vi "Create.vi"(8 "error in (no error)":errorcluster, 9 "Denumerator":i64=1, 10 "Numerator":i64) -> (0 "error out":errorcluster, 3 "Hi Res Arithm Test":refnum<class "High Res Arithmetic.lvclass">)   [LabVIEW 2021, in "High Res Arithmetic.lvclass"]
uses:
  High Res Arithmetic/High Res Arithmetic.lvclass
  High Res Arithmetic/High Res Arithmetic.lvclass/High Res Arithmetic.ctl
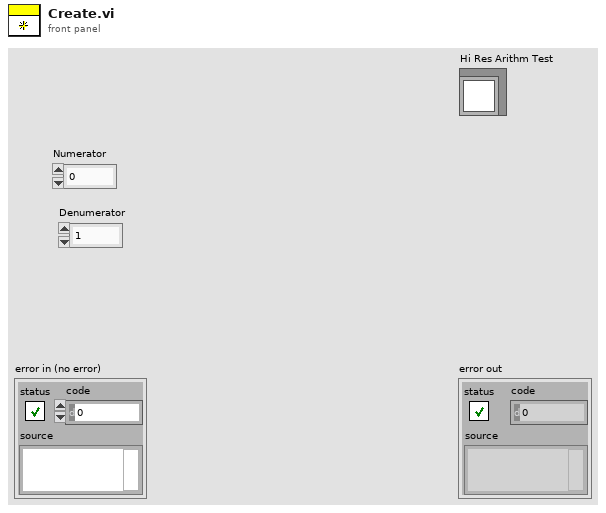
[diagram p1: front panel]
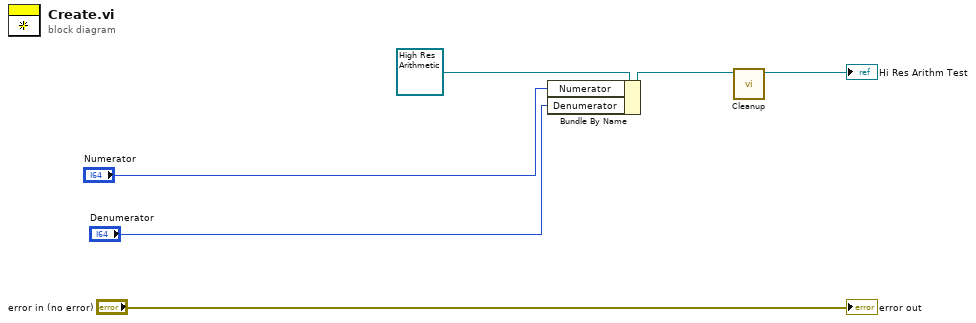
[diagram p0: block diagram]
diagram:
  n1 = Bundle By Name(cluster=refnum<class "High Res Arithmetic.lvclass"> refnum ("Hi Res Arithm Test"), "Numerator"="Numerator", "Denumerator"="Denumerator") -> (w4:refnum<class "High Res Arithmetic.lvclass">)
  n2 = call "Cleanup.vi"("High Res Arithmetic in"=w4) -> ("High Res Arithmetic out"=→"Hi Res Arithm Test":refnum<class "High Res Arithmetic.lvclass">)  [unwired: 9 in, 1 out]
  "error out" <- "error in (no error)"
